vi "WindowsMediaPlayer.vi"() -> ()   [LabVIEW 2011]
panel:
  in  "Load":bool
  in  "currentPosition":dbl
  in  "Path":path
  in  "WindowsMediaPlayer":refnum<k7>(container)
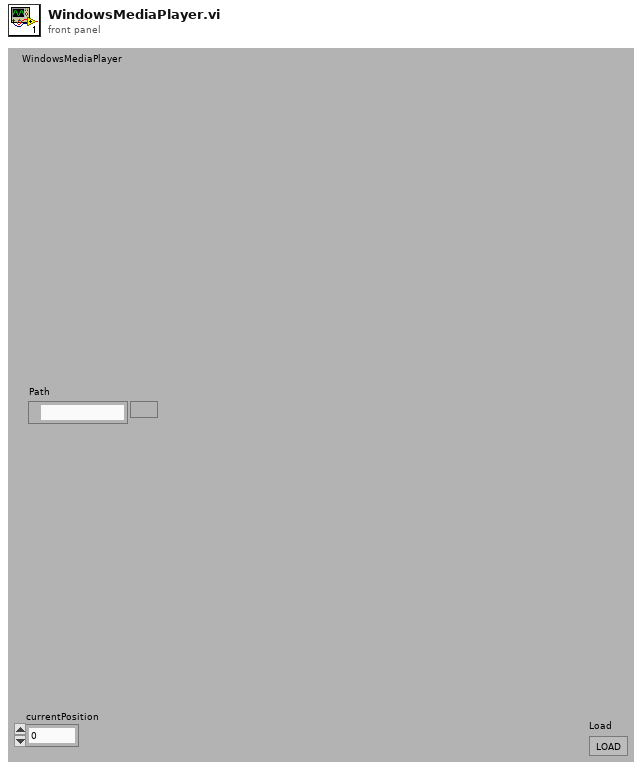
[diagram p1: front panel]
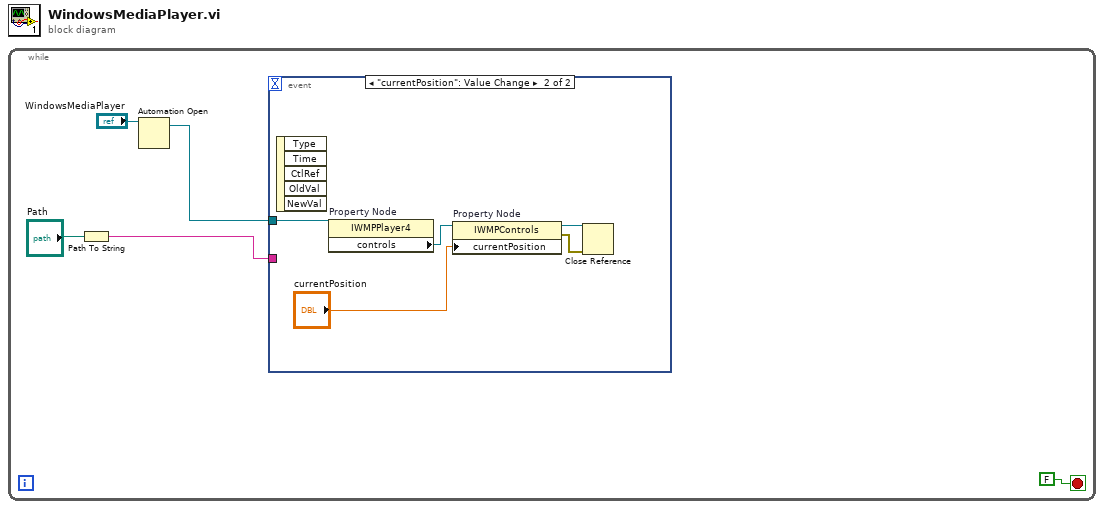
[diagram p0: block diagram]
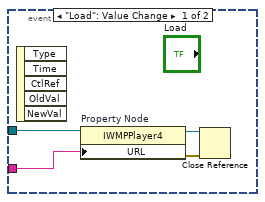
[diagram p2: hidden frame]
diagram:
  n1 = while {
    stop <- FALSE stop-if-true
    n2 = Path To String(path="Path") -> (string=w2:string)
    n3 = Automation Open(Automation Refnum="WindowsMediaPlayer") -> (Automation Refnum=w5:refnum<k7>)  [unwired: 1 in, 3 out]
    n4 = event shown="[1] \"currentPosition\": Value Change" {
      selector: _ -> [_ _]
      dyn-events: _ -> [_ _]
      timeout: _ -> [_ _]
      tunnel: w5 -> [w9 w14]
      tunnel: w2 -> [w8 _]
      event "Load": Value Change {
        n5 = event-data() -> ()  [unwired: 1 in, 5 out]
        n6 = property on="Property Node" class="IWMPPlayer4"(reference=w9, "URL"=w8) -> (reference out=w7:refnum<k7>, error out=w6:errorcluster)  [unwired: 1 in]
        n7 = Close Reference(reference=w7, error in (no error)=w6) -> ()  [unwired: 1 out]
      }
      event "currentPosition": Value Change {
        n8 = event-data() -> ()  [unwired: 1 in, 5 out]
        n9 = property on="Property Node" class="IWMPPlayer4"(reference=w14) -> ("controls"=w13:refnum<k7>)  [unwired: 1 in, 2 out]
        n10 = property on="Property Node" class="IWMPControls"(reference=w13, "currentPosition"="currentPosition") -> (reference out=w11:refnum<k7>, error out=w10:errorcluster)  [unwired: 1 in]
        n11 = Close Reference(reference=w11, error in (no error)=w10) -> ()  [unwired: 1 out]
      }
    }
  }
